vi "GroupShuffleSplit.vi"(6 "Groups":string[][](array[string]), 8 "error in (no error)":errorcluster caption="entrée d'erreur (pas d'erreur)", 9 "y":string[][](array[string]), 10 "X":string[][](array[string]), 11 "GroupShuffleSplit":T2={"n_splits"=5, "test_size"="0,2", "train_size"="None", "random_state"=-1} {"random_state" min=-1}) -> (0 "error out":errorcluster caption="sortie d'erreur", 3 "Split":T1(array[cluster]))   [LabVIEW 2020]
doc: "Shuffle-Group(s)-Out cross-validation iterator\n\nProvides randomized train/test indices to split data according to a third-party provided group. This group information can be used to encode arbitrary domain specific stratifications of the samples as integers.\n\nFor instance the groups could be the year of collection of the samples and thus allow for cross-validation against time-based splits.\n\nThe difference between LeavePGroupsOut and GroupShuffleSplit is that the former generates splits using all subsets of size p unique groups, whereas GroupShuffleSplit generates a user-determined number of random test splits, each with a user-determined fraction of unique groups.\n\nFor example, a less computationally intensive alternative to LeavePGroupsOut(p=10) would be GroupShuffleSplit(test_size=10, n_splits=100).\n\nNote: The parameters test_size and train_size refer to groups, and not to samples, as in ShuffleSplit.\n\n\n\nParameters : \n\n- n_splits : int, default=5\nNumber of re-shuffling & splitting iterations.\n\n- test_size : float, int, default=0.2\nIf float, should be between 0.0 and 1.0 and represent the proportion of groups to include in the test split (rounded up). If int, represents the absolute number of test groups. If None, the value is set to the complement of the train size. The default will change in version 0.21. It will remain 0.2 only if train_size is unspecified, otherwise it will complement the specified train_size.\n\n- train_size : float or int, default=None\nIf float, should be between 0.0 and 1.0 and represent the proportion of the groups to include in the train split. If int, represents the absolute number of train groups. If None, the value is automatically set to the complement of the test size.\n\n- random_state : int or RandomState instance, default=None=-1\nControls the randomness of the training and testing indices produced. Pass an int for reproducible output across multiple function calls. See Glossary.\n\n\nMethods : Split\n\n\nParameters : \n\n- X : array-like of shape (n_samples, n_features)\nTraining data, where n_samples is the number of samples and n_features is the number of features.\n\n- y : array-like of shape (n_samples,), default=None\nThe target variable for supervised learning problems.\n\n- groups : array-like of shape (n_samples,)\nGroup labels for the samples used while splitting the dataset into train/test set.\n\nYields :\n \n- train : ndarray\nThe training set indices for that split.\n\n- test : ndarray\nThe testing set indices for that split."
uses:
  GroupShuffleSplit.lvclass
panel:
  out "GroupShuffleSplit.lvclass":refnum<class "GroupShuffleSplit.lvclass">
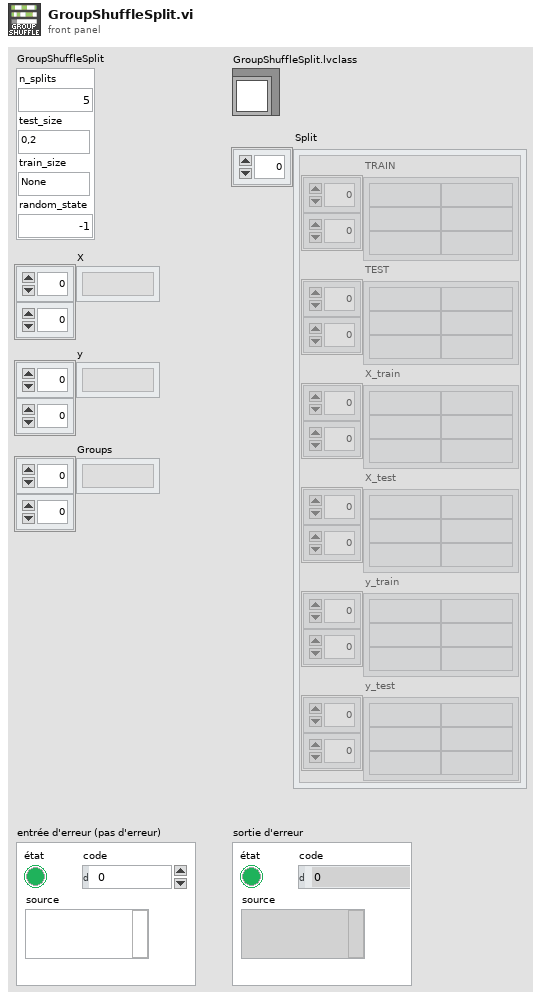
[diagram p1: front panel]
types:
  T1 = cluster{"TRAIN":string[][], "TEST":string[][], "X_train":string[][], "X_test":string[][], "y_train":string[][], "y_test":string[][]}[]
  T2 = cluster{"n_splits":i32, "test_size":string, "train_size":string, "random_state":i32}
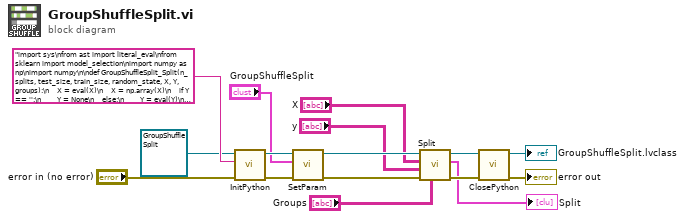
[diagram p0: block diagram]
diagram:
  n1 = call-dynamic "InitPython.vi"("error in (no error)"="error in (no error)", "Python Instruction"="import sys\nfrom ast import literal_eval\nfrom sklearn import model_selection\nimport numpy as np\nimport numpy\n\ndef GroupShuffleSplit_Split(n_splits, test_size, train_size, random_state, X, Y, groups):\n    X = eval(X)\n    X = np.array(X)\n    if Y == '':\n        Y = None\n    else:\n        Y = eval(Y)\n        Y = np.array(Y)\n    if groups == '':\n        groups = None\n    else:\n        groups = eval(groups)\n        groups = np.array(groups)\n    if test_size == 'None':\n        test_size = None\n    else:\n         test_size = eval(test_size)\n    if train_size == 'None':\n        train_size = None\n    else:\n         train_size = eval(train_size)\n    if random_state == -1:\n        random_state = None\n    list_return = []\n    try:\n        for train_index, test_index in model_selection.GroupShuffleSplit(n_splits, test_size, train_size, random_state).split(X, Y, groups):\n            list_return = list_return +[\"TRAIN:\", train_index.tolist(), \"TEST:\", test_index.tolist()]\n            X_train, X_test = X[train_index].tolist(), X[test_index].tolist()\n            y_train, y_test = Y[train_index].tolist(), Y[test_index].tolist()\n            list_return = list_return +[\"X_train:\", X_train, \"X_test:\", X_test, \"y_train:\", y_train, \"y_test:\", y_test]\n        return str(list_return)\n    except:\n        erreur = sys.exc_info()\n        typerr = u\"%s\" % (erreur[0])\n        typerr = typerr[typerr.find(\"'\")+1:typerr.rfind(\"'\")]\n        msgerr = u\"%s\" % (erreur[1])\n        message = str('/!\\\\ {0} : {1}'. format(typerr,msgerr))\n        return message", "Scikit-learn en entrée"=refnum<class "GroupShuffleSplit.lvclass"> refnum ("GroupShuffleSplit.lvclass")) -> ("error out"=w13:errorcluster, "Scikit-learn en sortie"=w12:refnum<class "GroupShuffleSplit.lvclass">)  [unwired: 7 in]
  n2 = call-dynamic "SetParam.vi"("error in (no error)"=w13, "GroupShuffleSplit"="GroupShuffleSplit", "GroupShuffleSplit.lvclass"=w12) -> ("error out"=w10:errorcluster, "GroupShuffleSplit.lvclass"=w9:refnum<class "GroupShuffleSplit.lvclass">)  [unwired: 7 in]
  n3 = call-dynamic "Split.vi"("Groups"="Groups", "error in (no error)"=w10, "y"="y", "X"="X", "GroupShuffleSplit.lvclass"=w9) -> ("error out"=w8:errorcluster, "Split"=→"Split":T1, "GroupShuffleSplit.lvclass"=w7:refnum<class "GroupShuffleSplit.lvclass">)  [unwired: 4 in]
  n4 = call-dynamic "ClosePython.vi"("error in (no error)"=w8, "Scikit-learn en entrée"=w7) -> ("error out"=→"error out":errorcluster, "Scikit-learn en sortie"=→"GroupShuffleSplit.lvclass":refnum<class "GroupShuffleSplit.lvclass">)  [unwired: 8 in]
